vi "API.vi"() -> ()   [LabVIEW 2018]
uses:
  7eaf2191-3900-4e37-b8f1-0b56292f964b.vi
  b105d130-1003-4e1c-a69e-171ed3b4cd62.vi
  164712d4-a40f-4c1d-9dd6-f0e909c7f9ac.vi
  f83999bd-597e-49a3-8a24-f514c2e803fa.vi
  e2d3a09e-3eda-43e4-847b-f5ba23d2d1dd.vi
  ef0be5a8-4980-411d-972c-ca998a3188ce.vi
  0dfa3e82-4891-44d4-bf0f-fa00f786f96a.vi
  bb7e9841-758c-4434-a6dd-f489ab997295.vi
  83cdd324-15c3-40f2-bb86-434760b938a2.vi
  6536fed6-d68e-4967-8e6a-e2def0745587.vi
  d3567d77-016b-4747-ae39-8267dda81e1a.vi
  6fa4e6d2-d40c-4a7c-8a57-a21af05c07b8.vi
  6ff51e3a-8f52-4f4b-8c43-8d4f807ed1ff.vi
  9bf46c02-7a8f-4e83-8ee1-f8cedbfdb624.vi
  27b3211a-0c0d-41bc-ab24-ed8bc60d9a3e.vi
  3f72ac97-b943-4619-9f88-611e59474e32.vi
  a345b58e-fa81-498b-941c-1bfe72ced7b2.vi
  62821ff5-7b51-4fb3-8449-2ccbb7cfd9cf.vi
  72defa96-1dad-4704-b983-8c3a2842dd53.vi
  c5faf44e-6c66-4be6-bc49-170f88b0dffb.vi
  8ea95075-ec7b-4070-b8fa-2f3b772012e4.vi
  dd124b5f-36c7-4e7c-bcc8-37bfffb7cae4.vi
  e474f224-f7a3-43aa-a45f-3a67769dfe2a.vi
  07250549-d10d-456d-a904-2844bfcc495d.vi
  ae986f24-a7ff-4199-9233-b7b7c6968880.vi
  9e916d3a-5ac6-4fc2-a2fa-7fe4c15454f8.vi
  7aebeb67-ab8c-4713-bde1-9c17d4f11bef.vi
  6ef498ff-9a86-45fa-8117-a9feb7d14522.vi
  4e4e8436-cb8d-404f-82fa-ebc67d0ba01b.vi
  0639858e-36a1-4160-b0c8-2a1ecd9bc163.vi
  fa3684de-dde7-447b-a0c7-f9517c264816.vi
  a08bfecc-65b3-42ab-aaa1-4bc22297f789.vi
  36e664cb-fb6c-47e5-b2de-b7d00e2e4ce9.vi
  41c6ab6b-5887-493e-861c-45756cbf9d42.vi
  3327472a-e7dc-4860-903c-8adc20d67148.vi
  9c7a3ae1-6096-40d8-8e14-c579b6ed278c.vi
  7cb3ad25-921b-421a-b41a-040235a55a67.vi
  4be9d3d4-5d57-462c-b657-92f67c871d92.vi
  e975bbf4-9770-493d-bfef-743597d641e8.vi
  144b26b2-e6d7-4242-9194-bbdb4e562a7b.vi
  api/GLog.lvlib
panel:
  out "double out":dbl format="%.2f"
  out "integer out":i32
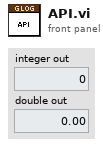
[diagram p1: front panel]
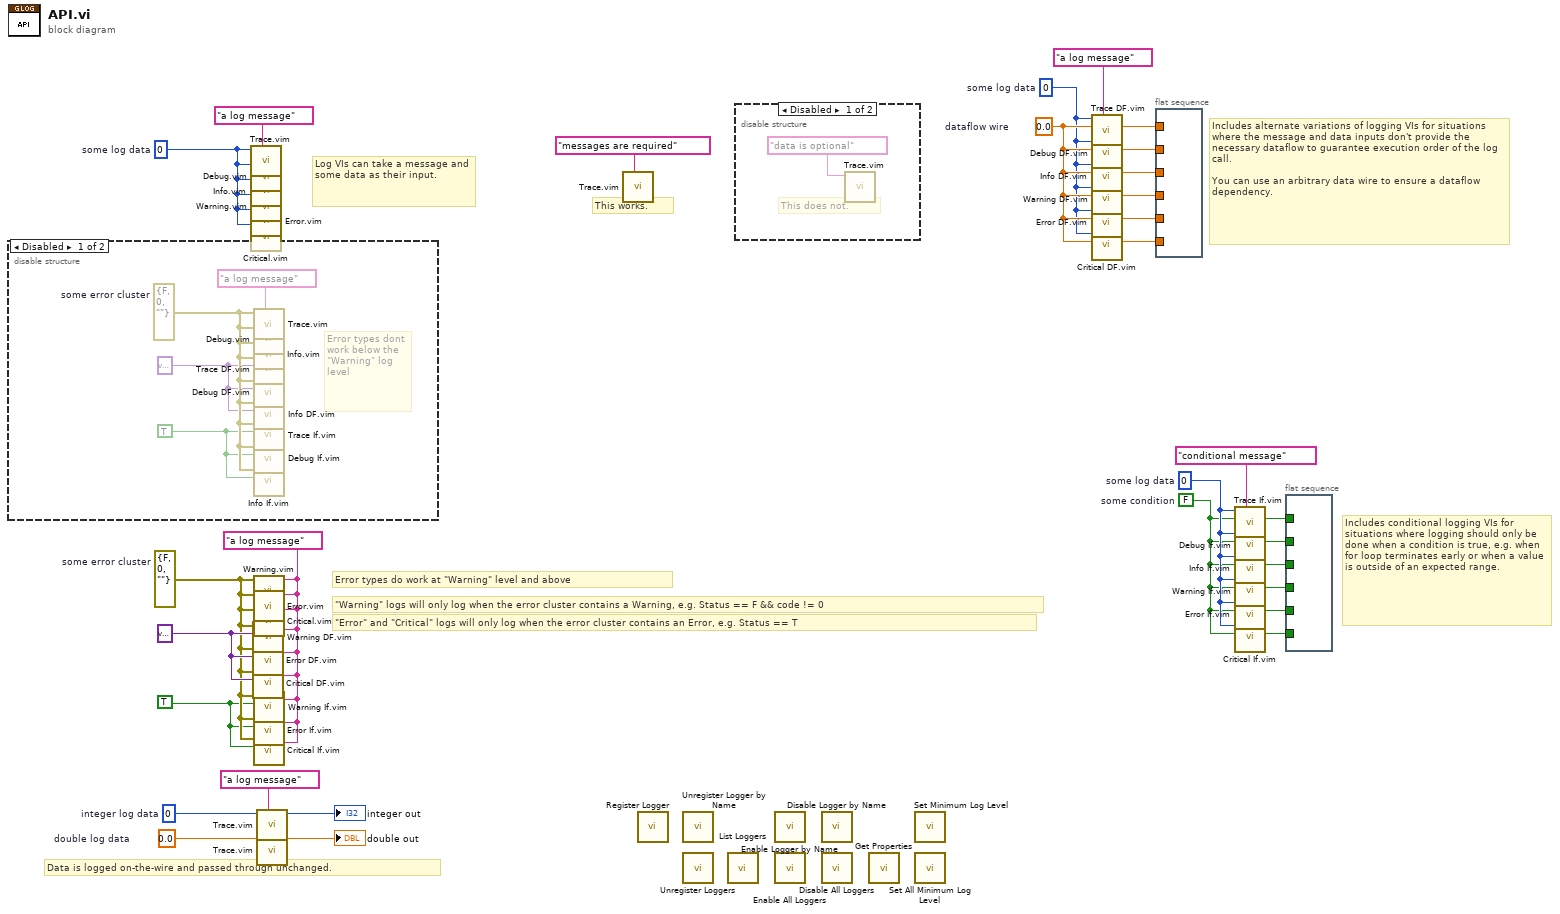
[diagram p0: block diagram]
diagram:
  w1 = TRUE
  w4 = variant
  w11 = FALSE  # some condition
  w12 = 0  # some log data
  w13 = "conditional message"
  w19 = 0.0  # dataflow wire
  w22 = "a log message"
  w14 = 0  # some log data
  w25 = 0.0  # double log data
  w28 = 0  # integer log data
  w24 = "a log message"
  w3 = "a log message"
  w2 = errorcluster {"status"=FALSE, "code"=0, "source"=""}  # some error cluster
  w29 = 0  # some log data
  w30 = "a log message"
  # "Includes conditional logging VIs for situations where logging should only be done when a condition is true, e.g. when for loop terminates early or when a value is outside of an expected range."
  # "\"Error\" and \"Critical\" logs will only log when the error cluster contains an Error, e.g. Status == T"
  # "\"Warning\" logs will only log when the error cluster contains a Warning, e.g. Status == F && code != 0"
  # "Includes alternate variations of logging VIs for situations where the message and data inputs don't provide the necessary dataflow to guarantee execution order of the log call.\n\nYou can use an arbitrary data wire to ensure a dataflow dependency."
  # "This works."
  # "Log VIs can take a message and some data as their input."
  # "Data is logged on-the-wire and passed through unchanged."
  # "Error types do work at \"Warning\" level and above"
  n1 = disable-structure shown="Disabled" {
    frame Disabled {
      w31 = TRUE
      w32 = variant
      w33 = errorcluster {"status"=FALSE, "code"=0, "source"=""}  # some error cluster
      w34 = "a log message"
      # "Error types dont work below the \"Warning\" log level"
      n2 = call "Trace.vim"("data in (null)"=w33, "message"=w34) -> ()  [unwired: 9 in, 1 out]
      n3 = call "Debug.vim"("data in (null)"=w33, "message"=w34) -> ()  [unwired: 9 in, 1 out]
      n4 = call "Info.vim"("data in (null)"=w33, "message"=w34) -> ()  [unwired: 9 in, 1 out]
      n5 = call "Trace DF.vim"("message"=w34, "dataflow in"=w32, "data (null)"=w33) -> ()  [unwired: 8 in, 1 out]
      n6 = call "Debug DF.vim"("message"=w34, "dataflow in"=w32, "data (null)"=w33) -> ()  [unwired: 8 in, 1 out]
      n7 = call "Info DF.vim"("message"=w34, "dataflow in"=w32, "data (null)"=w33) -> ()  [unwired: 8 in, 1 out]
      n8 = call "Trace If.vim"("message"=w34, "condition in"=w31, "data (null)"=w33) -> ()  [unwired: 8 in, 1 out]
      n9 = call "Debug If.vim"("message"=w34, "condition in"=w31, "data (null)"=w33) -> ()  [unwired: 8 in, 1 out]
      n10 = call "Info If.vim"("message"=w34, "condition in"=w31, "data (null)"=w33) -> ()  [unwired: 8 in, 1 out]
    }
    frame Enabled {
    }
  }
  n11 = call "Trace.vim"("data in (null)"=w29, "message"=w30) -> ()  [unwired: 9 in, 1 out]
  n12 = call "Debug.vim"("data in (null)"=w29, "message"=w30) -> ()  [unwired: 9 in, 1 out]
  n13 = call "Info.vim"("data in (null)"=w29, "message"=w30) -> ()  [unwired: 9 in, 1 out]
  n14 = call "Warning.vim"("data in (null)"=w29, "message"=w30) -> ()  [unwired: 9 in, 1 out]
  n15 = call "Error.vim"("data in (null)"=w29, "message"=w30) -> ()  [unwired: 9 in, 1 out]
  n16 = call "Critical.vim"("data in (null)"=w29, "message"=w30) -> ()  [unwired: 9 in, 1 out]
  n17 = call "Warning DF.vim"("message"=w3, "dataflow in"=w4, "data (null)"=w2) -> ()  [unwired: 8 in, 1 out]
  n18 = call "Error DF.vim"("message"=w3, "dataflow in"=w4, "data (null)"=w2) -> ()  [unwired: 8 in, 1 out]
  n19 = call "Critical DF.vim"("message"=w3, "dataflow in"=w4, "data (null)"=w2) -> ()  [unwired: 8 in, 1 out]
  n20 = call "Warning.vim"("data in (null)"=w2, "message"=w3) -> ()  [unwired: 9 in, 1 out]
  n21 = call "Error.vim"("data in (null)"=w2, "message"=w3) -> ()  [unwired: 9 in, 1 out]
  n22 = call "Critical.vim"("data in (null)"=w2, "message"=w3) -> ()  [unwired: 9 in, 1 out]
  n23 = call "Warning If.vim"("message"=w3, "condition in"=w1, "data (null)"=w2) -> ()  [unwired: 8 in, 1 out]
  n24 = call "Error If.vim"("message"=w3, "condition in"=w1, "data (null)"=w2) -> ()  [unwired: 8 in, 1 out]
  n25 = call "Critical If.vim"("message"=w3, "condition in"=w1, "data (null)"=w2) -> ()  [unwired: 8 in, 1 out]
  n26 = call "Trace.vim"("data in (null)"=w28, "message"=w24) -> ("data out"=→"integer out":i32)  [unwired: 9 in]
  n27 = call "Trace.vim"("data in (null)"=w25, "message"=w24) -> ("data out"=→"double out":dbl)  [unwired: 9 in]
  n28 = call "Trace.vim"("message"="messages are required") -> ()  [unwired: 10 in, 1 out]
  n29 = call "Register Logger.vi"() -> ()  [unwired: 11 in, 1 out]
  n30 = call "Unregister Logger by Name.vi"() -> ()  [unwired: 10 in, 2 out]
  n31 = call "Unregister Loggers.vi"() -> ()  [unwired: 10 in, 2 out]
  n32 = call "List Loggers.vi"() -> ()  [unwired: 10 in, 2 out]
  n33 = disable-structure shown="Disabled" {
    frame Disabled {
      # "This does not."
      n34 = call "Trace.vim"("data in (null)"="data is optional") -> ()  [unwired: 10 in, 1 out]
    }
    frame Enabled {
    }
  }
  n35 = call "Enable Logger by Name.vi"() -> ()  [unwired: 11 in, 1 out]
  n36 = call "Enable All Loggers.vi"() -> ()  [unwired: 11 in, 1 out]
  n37 = call "Disable Logger by Name.vi"() -> ()  [unwired: 11 in, 1 out]
  n38 = call "Disable All Loggers.vi"() -> ()  [unwired: 11 in, 1 out]
  n39 = call "Get Properties.vi"() -> ()  [unwired: 10 in, 2 out]
  n40 = call "Set Minimum Log Level.vi"() -> ()  [unwired: 11 in, 1 out]
  n41 = call "Set All Minimum Log Level.vi"() -> ()  [unwired: 11 in, 1 out]
  n42 = call "Trace DF.vim"("message"=w22, "dataflow in"=w19, "data (null)"=w14) -> ("dataflow out"=w21:dbl)  [unwired: 8 in]
  n43 = call "Debug DF.vim"("message"=w22, "dataflow in"=w19, "data (null)"=w14) -> ("dataflow out"=w20:dbl)  [unwired: 8 in]
  n44 = call "Info DF.vim"("message"=w22, "dataflow in"=w19, "data (null)"=w14) -> ("dataflow out"=w18:dbl)  [unwired: 8 in]
  n45 = call "Warning DF.vim"("message"=w22, "dataflow in"=w19, "data (null)"=w14) -> ("dataflow out"=w17:dbl)  [unwired: 8 in]
  n46 = call "Error DF.vim"("message"=w22, "dataflow in"=w19, "data (null)"=w14) -> ("dataflow out"=w16:dbl)  [unwired: 8 in]
  n47 = call "Critical DF.vim"("message"=w22, "dataflow in"=w19, "data (null)"=w14) -> ("dataflow out"=w15:dbl)  [unwired: 8 in]
  n48 = flat-sequence {
    tunnel: w21 -> [_]
    tunnel: w20 -> [_]
    tunnel: w18 -> [_]
    tunnel: w17 -> [_]
    tunnel: w16 -> [_]
    tunnel: w15 -> [_]
    frame #0 {
    }
  }
  n49 = call "Trace If.vim"("message"=w13, "condition in"=w11, "data (null)"=w12) -> ("condition out"=w10:bool)  [unwired: 8 in]
  n50 = call "Debug If.vim"("message"=w13, "condition in"=w11, "data (null)"=w12) -> ("condition out"=w9:bool)  [unwired: 8 in]
  n51 = call "Info If.vim"("message"=w13, "condition in"=w11, "data (null)"=w12) -> ("condition out"=w8:bool)  [unwired: 8 in]
  n52 = call "Warning If.vim"("message"=w13, "condition in"=w11, "data (null)"=w12) -> ("condition out"=w7:bool)  [unwired: 8 in]
  n53 = call "Error If.vim"("message"=w13, "condition in"=w11, "data (null)"=w12) -> ("condition out"=w6:bool)  [unwired: 8 in]
  n54 = call "Critical If.vim"("message"=w13, "condition in"=w11, "data (null)"=w12) -> ("condition out"=w5:bool)  [unwired: 8 in]
  n55 = flat-sequence {
    tunnel: w10 -> [_]
    tunnel: w9 -> [_]
    tunnel: w8 -> [_]
    tunnel: w7 -> [_]
    tunnel: w6 -> [_]
    tunnel: w5 -> [_]
    frame #0 {
    }
  }
